vi "Write String.vi"(7 "Channel Name":string, 8 "error in (no error)":errorcluster, 9 "Data Value":dbl, 10 "Bus In":refnum<class "Bus.lvclass">, 11 "NI Digital in":refnum<class "String Out.lvclass">) -> (0 "error out":errorcluster, 2 "Bus Out":refnum<class "Bus.lvclass">, 3 "NI Digital out":refnum<class "String Out.lvclass">)   [LabVIEW 2018, in "String Out.lvclass"]
doc: "String Out.lvclass:Read String.vi\n\nThis is the template for the Read String VI forthe String Out class.\n\nInstrument Communication Module Version 1.0\nOctober, 2020 Original Code Consulting Davita Bird\n www.originalcode.com"
uses:
  String Out.lvclass
  Bus/Bus.lvclass
  String Out.lvclass/String Out.ctl
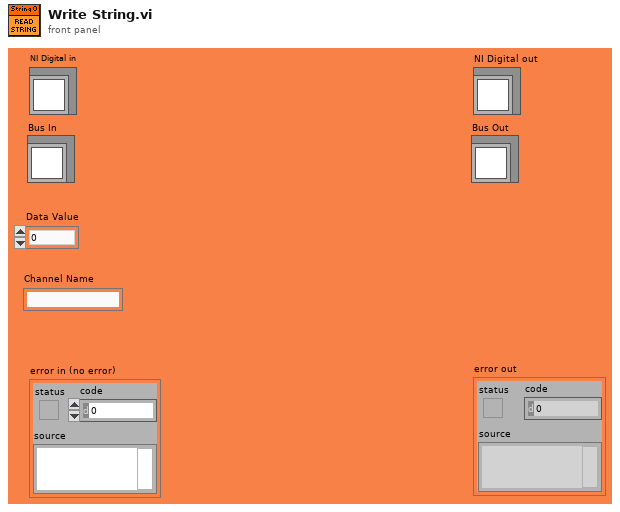
[diagram p1: front panel]
types:
  T1 = cluster{"String":string, "Replacement String":string}[]
  T2 = cluster{"String":string, "Replacement String":string}
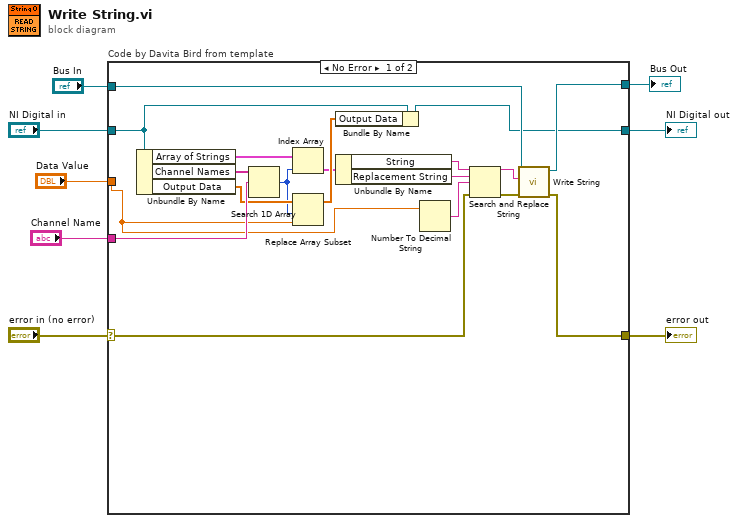
[diagram p0: block diagram]
diagram:
  n1 = case "Code by Davita Bird from template" shown="No Error" "error in (no error)" {
    selector: "error in (no error)" -> [w23 w30]
    tunnel: [w24 w30] -> w7
    tunnel: [w19 w29] -> w6
    tunnel: "NI Digital in" -> [w27 w29]
    tunnel: "Data Value" -> [w15 _]
    tunnel: "Bus In" -> [w25 w28]
    tunnel: [w26 w28] -> w3
    tunnel: "Channel Name" -> [w17 _]
    frame No Error {
      n2 = Unbundle By Name(w27) -> ("Array of Strings"=w13:T1, "Channel Names"=w18:string[], "Output Data"=w16:dbl[])
      n3 = Search 1D Array(1D array=w18, element=w17) -> (index of element=w12:i32)  [unwired: 1 in]
      n4 = Index Array(array=w13, index=w12) -> (element=w11:T2)
      n5 = Replace Array Subset(array=w16, new element=w15, index=w12) -> (w14:dbl[])
      n6 = Bundle By Name(cluster=w27, "Output Data"=w14) -> (w19:refnum<class "String Out.lvclass">)
      n7 = Unbundle By Name(w11) -> ("String"=w10:string, "Replacement String"=w9:string)
      n8 = Number To Decimal String(number=w15) -> (decimal integer string=w20:string)  [unwired: 1 in]
      n9 = Search and Replace String(input string=w10, search string=w9, replace string=w20, error in=w23) -> (result string=w21:string, error out=w22:errorcluster)  [unwired: 4 in, 2 out]
      n10 = call-dynamic "Write String.vi"("error in (no error)"=w22, "String"=w21, "Bus in"=w25) -> ("error out"=w24:errorcluster, "Bus out"=w26:refnum<class "Bus.lvclass">)  [unwired: 7 in]
    }
    frame Error {
    }
  }
  "error out" <- w7
  "NI Digital out" <- w6
  "Bus Out" <- w3
